vi "capturingSpectImage.vi"(8 "error in (no error)":errorcluster, 9 "command_captureSpectImage":T1, 10 "model in":refnum<class "IModel.lvclass">, 11 "CapturingSpectImage in":refnum<class "CapturingSpectImageState.lvclass">) -> (0 "error out":errorcluster, 1 "Status":string, 2 "model out":refnum<class "IModel.lvclass">, 3 "CapturingSpectImage out":refnum<class "CapturingSpectImageState.lvclass">)   [LabVIEW 2016, in "States.lvlib" / "CapturingSpectImageState.lvclass"]
uses:
  CapturingSpectImageState.lvclass
  IModel/IModel.lvclass
  ts_sallv_sedspectrometer/DataTypes/command_captureSpectImage.ctl
  Typedefs/CommandValue.ctl
  Typedefs/SEDSpectrometerTypedefs.lvlib
  ts_sallv_sedspectrometer/SALLV_sedSpectrometer.lvlib
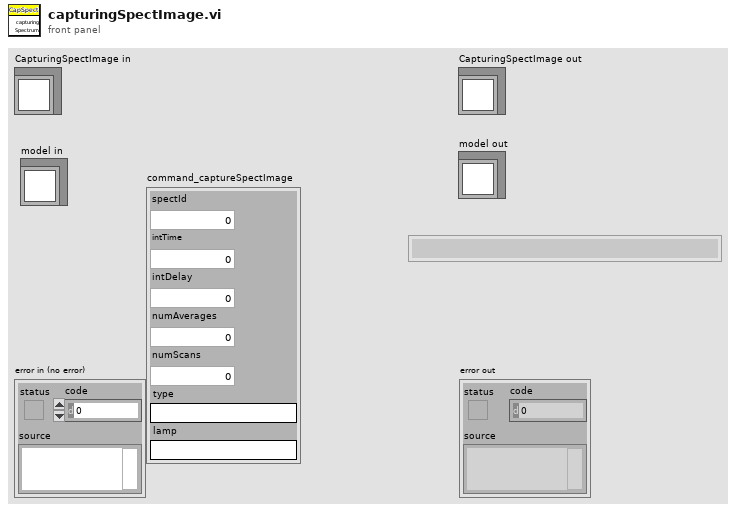
[diagram p1: front panel]
types:
  T1 = typedef "SALLV_sedSpectrometer.lvlib/command_captureSpectImage.ctl" = cluster{"spectId":u16, "intTime":sgl, "intDelay":dbl, "numAverages":u16, "numScans":i32, "type":string, "lamp":string}
  T2 = typedef "SEDSpectrometerTypedefs.lvlib/CommandValue.ctl" = enum16{"disable", "enable", "exit", "GoToStandby", "OnHeartbeat", "OnIncomingMessagingError", "OnInterrupt", "start", "captureSpectImage", "setSpectTempSetpoint", "stopImageCapture"}
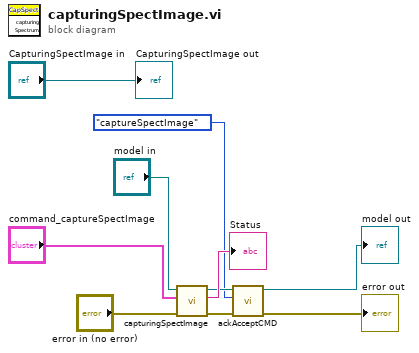
[diagram p0: block diagram]
diagram:
  n1 = call-dynamic "capturingSpectImage.vi"("error in (no error)"="error in (no error)", "command_captureSpectImage"="command_captureSpectImage", "IModel in"="model in") -> ("error out"=w3:errorcluster, "Status"=→"Status":string, "IModel out"=w5:refnum<class "IModel.lvclass">)  [unwired: 6 in]
  n2 = call-dynamic "ackAcceptCMD.vi"("error in (no error)"=w3, "CommandValue"=CommandValue."captureSpectImage", "IModel in"=w5) -> ("error out"=→"error out":errorcluster, "IModel out"=→"model out":refnum<class "IModel.lvclass">)  [unwired: 7 in]
  "CapturingSpectImage out" <- "CapturingSpectImage in"
